vi "Initialize.vi"(4 "error in (no error)":errorcluster, 7 "logging":bool) -> (0 "error out":errorcluster, 1 "DeviceKey List":string[](array[string]), 2 "DeviceIOLib Out":refnum<k24>, 3 "CmdLib Out":refnum<k24>)   [LabVIEW 2009]
uses:
  C:/Code/Apps/Utilities/Picomotor/PicomotorApp/Install/Samples/LabVIEW/Mixed Devices/LabVIEW 2009/CmdLib8742.dll
  C:/Code/Apps/Utilities/Picomotor/PicomotorApp/Install/Samples/LabVIEW/Mixed Devices/LabVIEW 2009/DeviceIOLib.dll
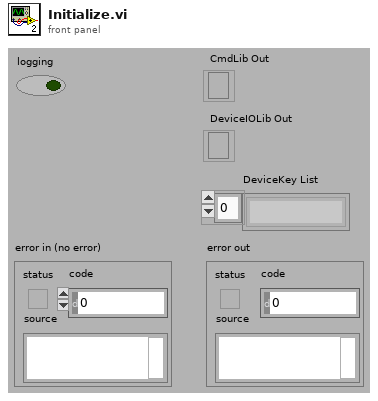
[diagram p1: front panel]
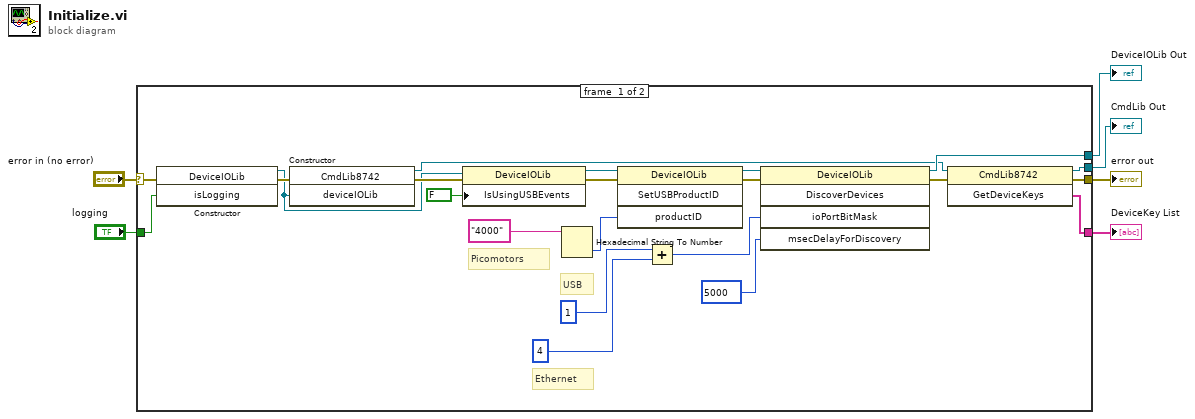
[diagram p0: block diagram]
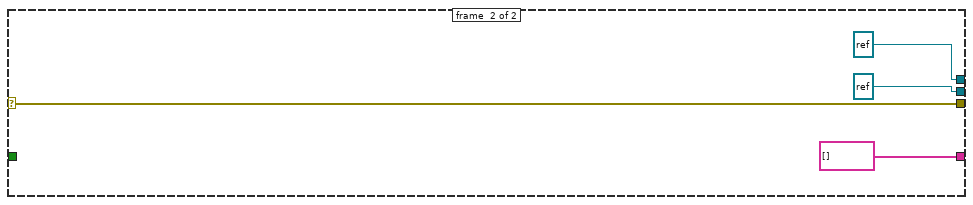
[diagram p2: hidden frame]
diagram:
  n1 = case shown="No Error" "error in (no error)" {
    selector: "error in (no error)" -> [w22 w32]
    tunnel: [w23 string[] [] ("GetDeviceKeys")] -> w6
    tunnel: [w21 w32] -> w4
    tunnel: [w16 refnum<k24> refnum ("new reference")] -> w3
    tunnel: "logging" -> [w20 _]
    tunnel: [w17 refnum<k24> refnum ("new reference")] -> w1
    frame #0 {
      # "Picomotors"
      # "Ethernet"
      # "USB"
      n2 = constructor class="DeviceIOLib"(error in=w22, "isLogging"=w20) -> (reference out=w10:refnum<k24>, error out=w12:errorcluster)  [unwired: 2 in, 2 out]
      n3 = constructor class="CmdLib8742"(error in=w12, "deviceIOLib"=w10) -> (reference out=w7:refnum<k24>, error out=w11:errorcluster)  [unwired: 2 in, 2 out]
      n4 = property class="DeviceIOLib"(reference=w10, error in=w11, "IsUsingUSBEvents"=FALSE) -> (reference out=w14:refnum<k24>, error out=w13:errorcluster)
      n5 = Hexadecimal String To Number(string="4000") -> (number=w19:u32)  [unwired: 2 in, 1 out]
      n6 = invoke class="DeviceIOLib" method="SetUSBProductID"(reference=w14, error in=w13, "productID"=w19) -> (reference out=w9:refnum<k24>, error out=w8:errorcluster)  [unwired: 1 in, 2 out]
      n7 = Add(x=1, y=4) -> (x+y=w24:i32)
      n8 = invoke class="DeviceIOLib" method="DiscoverDevices"(reference=w9, error in=w8, "ioPortBitMask"=w24, "msecDelayForDiscovery"=5000) -> (reference out=w17:refnum<k24>, error out=w15:errorcluster)  [unwired: 1 in, 3 out]
      n9 = invoke class="CmdLib8742" method="GetDeviceKeys"(reference=w7, error in=w15) -> (reference out=w16:refnum<k24>, error out=w21:errorcluster, "GetDeviceKeys"=w23:string[])  [unwired: 1 in]
    }
    frame #1 {
    }
  }
  "DeviceKey List" <- w6
  "error out" <- w4
  "CmdLib Out" <- w3
  "DeviceIOLib Out" <- w1
